vi "Write Last valid index.vi"(8 "error in (no error)":errorcluster, 10 "Last valid index":i32, 11 "parcour_Liste in":refnum<class "parcour_Liste.lvclass">) -> (0 "error out":errorcluster, 3 "parcour_Liste out":refnum<class "parcour_Liste.lvclass">)   [LabVIEW 2019, in "parcour_Liste.lvclass"]
uses:
  parcour_Liste.lvclass
  parcour_Liste.lvclass/parcour_Liste.ctl
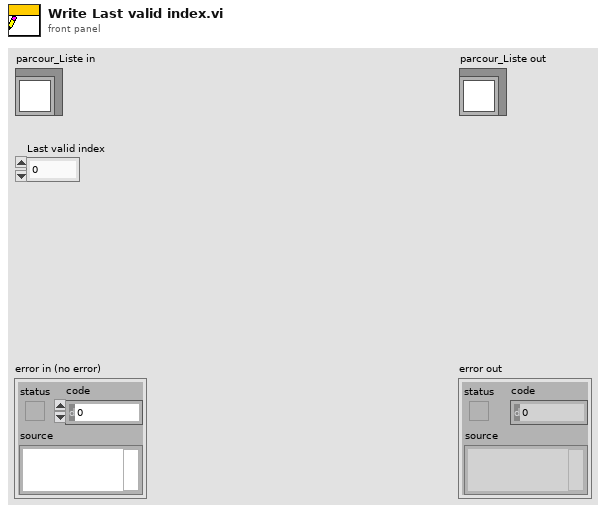
[diagram p1: front panel]
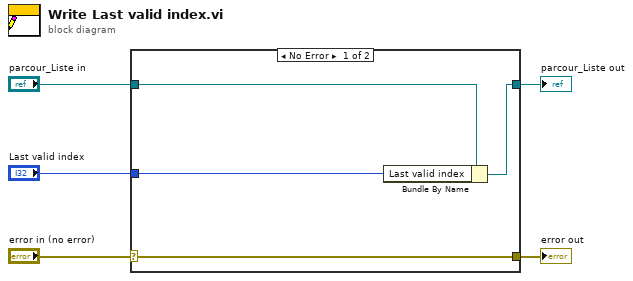
[diagram p0: block diagram]
diagram:
  n1 = case shown="No Error" "error in (no error)" {
    selector: "error in (no error)" -> [w9 w10]
    tunnel: [w9 w10] -> w4
    tunnel: [w7 w11] -> w2
    tunnel: "parcour_Liste in" -> [w8 w11]
    tunnel: "Last valid index" -> [w6 _]
    frame No Error {
      n2 = Bundle By Name(cluster=w8, "Last valid index"=w6) -> (w7:refnum<class "parcour_Liste.lvclass">)
    }
    frame Error {
    }
  }
  "error out" <- w4
  "parcour_Liste out" <- w2
